vi "TreeShrewPressureMeasurement.vi"() -> ()   [LabVIEW 2015]
uses:
  <vilib>/Utility/file.llb/Write To Spreadsheet File (DBL).vi
panel:
  out "max value":dbl
  out "Honeywell Pressure Transducer":dynamicdata(graph)
  in  "file path":path=path "C:/Users/Tonia/Desktop/Ocular Blast Data/Ocular Blast Pressure data.xls"
  in  "stop":bool
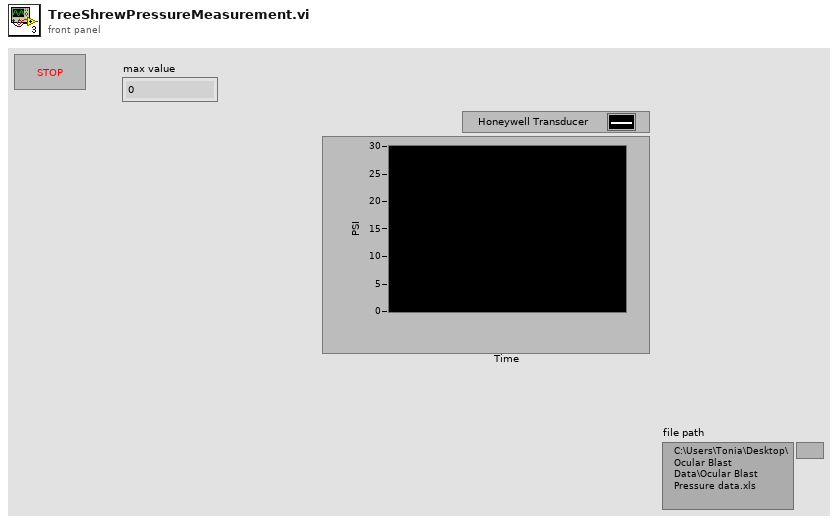
[diagram p1: front panel]
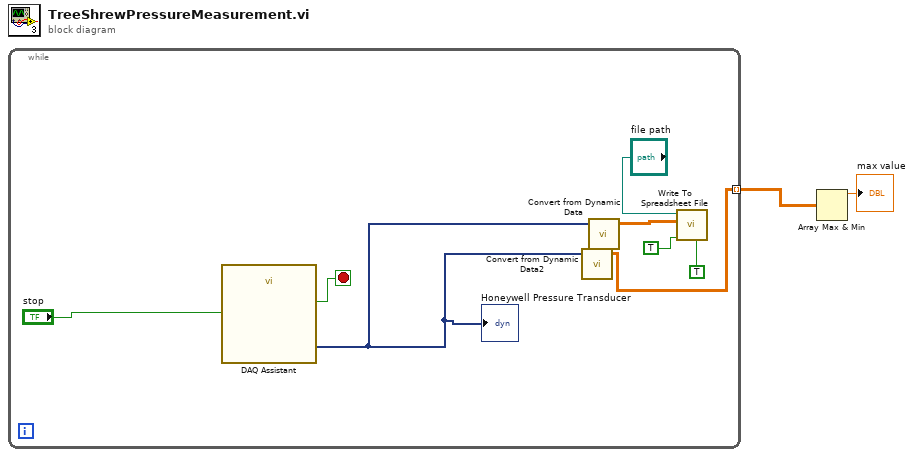
[diagram p0: block diagram]
diagram:
  n1 = while {
    tunnel: [w4] -> w2 mode=indexing
    stop <- w10 stop-if-true
    n2 = call "DAQ Assistant"("stop (F)"="stop") -> ("data"=w3:dynamicdata, "stopped"=w10:bool)  [unwired: 15 in, 2 out]
    "Honeywell Pressure Transducer" <- w3
    n3 = call "Convert from Dynamic Data2"("Dynamic Data Type"=w3) -> ("Array"=w4:dbl[][])  [unwired: 3 in]
    n4 = call "Convert from Dynamic Data"("Dynamic Data Type"=w3) -> ("Array"=w5:dbl[][])  [unwired: 3 in]
    n5 = call-poly <vilib>:"Write To Spreadsheet File.vi"("transpose? (no:F)"=TRUE, "append to file? (new file:F)"=TRUE, "2D data"=w5, "file path (dialog if empty)"="file path") -> ()  [unwired: 4 in, 1 out]
  }
  n6 = Array Max & Min(array=w2) -> (max value=→"max value":dbl)  [unwired: 3 out]
